vi "dotnet_event_callback.vi"(4 "Variant":variant, 5 "Event Data":cluster{"sender":refnum<k24>, "e":refnum<k24>}, 6 "Control Ref":refnum<k24>, 7 "Event Common Data":T1) -> ()   [LabVIEW 2017, in "BalloonNotifier.lvclass"]
uses:
  BalloonNotifier.lvclass
  balloon_NET_Callback_Parameter.ctl
  ballloon_user_event_ref.ctl
  balloon_event_data.ctl
  balloon_events.ctl
  System.Windows.Forms
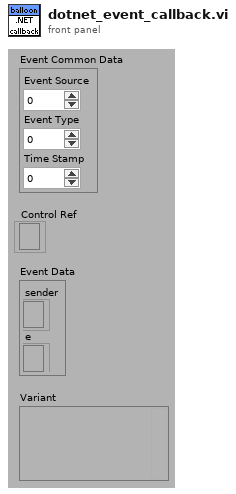
[diagram p1: front panel]
types:
  T1 = cluster{"Event Source":i32, "Event Type":u32, "Time Stamp":u32}
  T2 = typedef "BalloonNotifier.lvclass/balloon_events.ctl" = enum16{"BalloonTipClicked", "BalloonTipClosed", "BalloonTipShown", "Click", "Disposed", "DoubleClick", "MouseClick", "MouseDoubleClick", "MouseDown", "MouseMove", "MouseUp", "MenuItemClick", "MenuItemSelect"}
  T3 = typedef "BalloonNotifier.lvclass/balloon_event_data.ctl" = cluster{"NotifyIcon Event":T2, "Data String":string}
  T4 = typedef "BalloonNotifier.lvclass/balloon_NET_callback_parameter.ctl" = cluster{"NotifyIcon User Event Ref":T5, "Event Data":variant}
  T5 = typedef "BalloonNotifier.lvclass/ballloon_user_event_ref.ctl" = refnum<user-event>
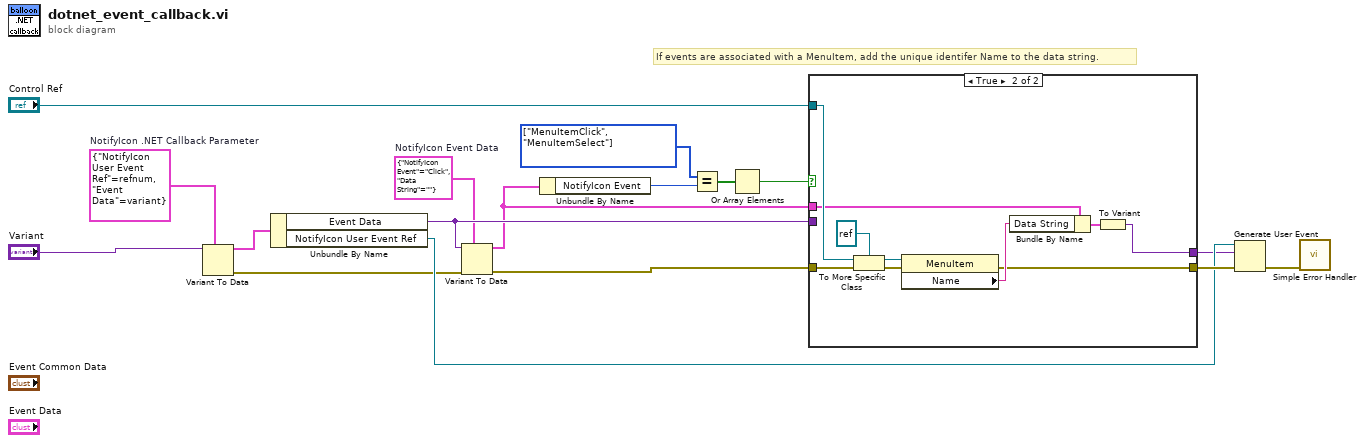
[diagram p0: block diagram]
diagram:
  w7 = T2[] [enum."MenuItemClick", enum."MenuItemSelect"] items=["BalloonTipClicked", "BalloonTipClosed", "BalloonTipShown", "Click", "Disposed", "DoubleClick", "MouseClick", "MouseDoubleClick", "MouseDown", "MouseMove", "MouseUp", "MenuItemClick", "MenuItemSelect"]
  w5 = T3 {"NotifyIcon Event"=enum."Click", "Data String"=""}  # NotifyIcon Event Data
  w4 = T4 {"NotifyIcon User Event Ref"=refnum, "Event Data"=variant}  # NotifyIcon .NET Callback Parameter
  # "If events are associated with a MenuItem, add the unique identifer Name to the data string."
  n1 = Variant To Data(type=w4, Variant="Variant") -> (data=w3:T4, error out=w11:errorcluster)  [unwired: 1 in]
  n2 = Unbundle By Name(w3) -> ("Event Data"=w15:variant, "NotifyIcon User Event Ref"=w16:T5)
  n3 = Variant To Data(error in=w11, type=w5, Variant=w15) -> (data=w13:T3, error out=w12:errorcluster)
  n4 = Unbundle By Name(w13) -> ("NotifyIcon Event"=w6:T2)
  n5 = Equal?(x=w7, y=w6) -> (x = y?=w8:bool[])
  n6 = Or Array Elements(Boolean array=w8) -> (logical OR=w9:bool)
  n7 = case shown="True" w9 {
    tunnel: "Control Ref" -> [_ w28]
    tunnel: w12 -> [w18 w27]
    tunnel: w13 -> [_ w24]
    tunnel: [w19 w21] -> w14
    tunnel: w15 -> [w19 _]
    tunnel: [w18 w20] -> w17
    frame False {
    }
    frame True {
      n8 = To More Specific Class(target class=refnum<k24> refnum ("reference"), reference=w28, error in=w27) -> (specific class reference=w26:refnum<k24>, error out=w25:errorcluster)
      n9 = property class="MenuItem"(reference=w26, error in=w25) -> (error out=w20:errorcluster, "Name"=w23:string)  [unwired: 1 out]
      n10 = Bundle By Name(cluster=w24, "Data String"=w23) -> (w22:T3)
      n11 = To Variant(anything=w22) -> (Variant=w21:variant)
    }
  }
  n12 = Generate User Event(user event=w16, event data cluster=w14, error in=w17) -> (error out=w2:errorcluster)  [unwired: 1 in, 1 out]
  n13 = call <vilib>:"Simple Error Handler.vi"("error in (no error)"=w2) -> ()  [unwired: 4 in, 5 out]
